vi "Set Defaults from Strings.vi"(8 "error in (no error)":errorcluster, 10 "Default Strings":string[](array[string]), 11 "GroupAbstract in":refnum<class "Group.lvclass">) -> (0 "error out":errorcluster, 3 "GroupAbstract out":refnum<class "Group.lvclass">)   [LabVIEW 2020, in "Vecto.lvlib" / "Group.lvclass"]
uses:
  Group.lvclass
  Group.lvclass/Group.ctl
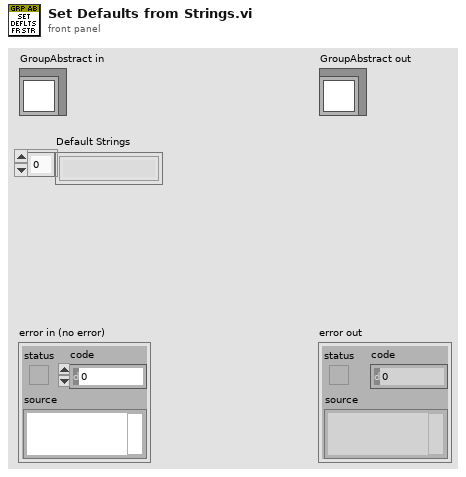
[diagram p1: front panel]
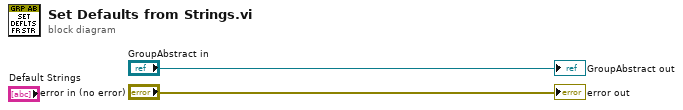
[diagram p0: block diagram]
diagram:
  "error out" <- "error in (no error)"
  "GroupAbstract out" <- "GroupAbstract in"
